vi "FileExists.vi"(1 "file path":path) -> (0 "Exists?":bool)   [LabVIEW 2014]
panel:
  out "error out":errorcluster
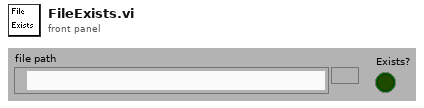
[diagram p1: front panel]
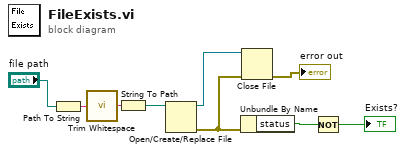
[diagram p0: block diagram]
diagram:
  n1 = Path To String(path="file path") -> (string=w3:string)
  n2 = call <vilib>:"Trim Whitespace.vi"("string"=w3) -> ("trimmed string"=w2:string)  [unwired: 1 in]
  n3 = String To Path(string=w2) -> (path=w1:path)
  n4 = Open/Create/Replace File(file path (use dialog)=w1) -> (refnum out=w7:refnum<file>, error out=w6:errorcluster)  [unwired: 5 in, 1 out]
  n5 = Unbundle By Name(w6) -> ("status"=w9:bool)
  n6 = Close File(refnum=w7, error in=w6) -> (error out=→"error out":errorcluster)  [unwired: 1 out]
  n7 = Not(x=w9) -> (.not. x?=→"Exists?":bool)
